vi "getScopeData.vi"(6 "TimeLabel":u32, 8 "error in (no error)":errorcluster, 9 "Spectrum":dbl[](array[numeric]), 10 "Device":i32, 11 "SEDSpectrometer in":refnum<class "SEDSpectrometer.lvclass">) -> (0 "error out":errorcluster, 1 "Spectrum":dbl[](array[numeric]), 2 "TimeLabel":u32, 3 "SEDSpectrometer out":refnum<class "SEDSpectrometer.lvclass">)   [LabVIEW 2016, in "SEDSpectrometer.lvclass"]
uses:
  SEDSpectrometer.lvclass
panel:
  out "Output Value":i32
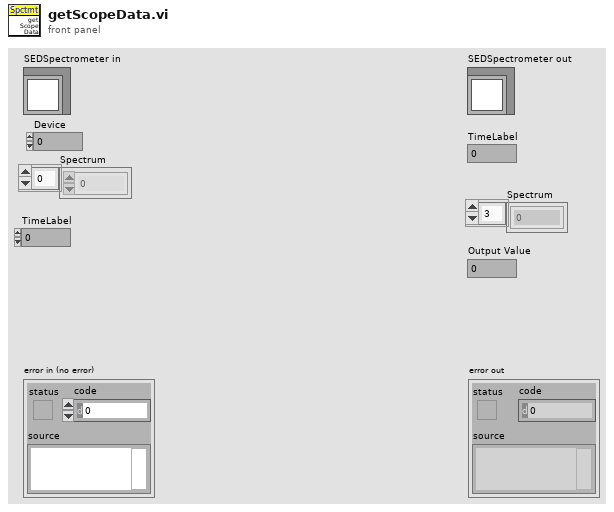
[diagram p1: front panel]
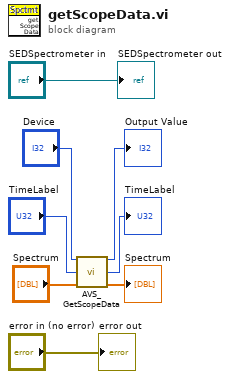
[diagram p0: block diagram]
diagram:
  n1 = call "AVS_GetScopeData.vi"("a_hDevice"="Device", "a_pTimeLabel"="TimeLabel", "a_pSpectrum"="Spectrum") -> ("Output Value"=→"Output Value":i32, "a_pTimeLabel"=→"TimeLabel":u32, "a_pSpectrum"=→"Spectrum":dbl[])  [unwired: 10 in]
  "error out" <- "error in (no error)"
  "SEDSpectrometer out" <- "SEDSpectrometer in"
